vi "SCLN_Servers.vi"() -> (0 "Number of Servers":i32=1 min=1 max=7)   [LabVIEW 2015]
doc: "This VI activates as many servers as declared in the \ninitialization VI. A listener for each server is created\nand a server loop is entered to handle the client\nmessages."
uses:
  SCLN_RW_Select.ctl
  SCLN_INT32_Select.ctl
  SCLN_NOTIF_Select.ctl
panel:
  out "Port7":string
  out "Port6":string
  out "Port5":string
  out "Port4":string
  out "Port3":string
  out "Port2":string
  out "Port1":string
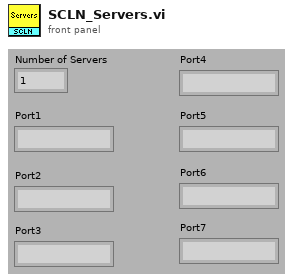
[diagram p1: front panel]
types:
  T1 = typedef "SCLN_INT32_Select.ctl" = enum16{"Max_Servers", "Max_Clients", "Total_Servers", "Total_Clients"}
  T2 = typedef "SCLN_RW_Select.ctl" = enum16{"Read", "Write"}
  T3 = typedef "SCLN_NOTIF_Select.ctl" = enum16{"Server1", "Server2", "Server3", "Server4", "Server5", "Server6", "Server7", "Client1", "Client2", "Client3", "Client4", "Client5", "Client6", "Client7", "Client8", "Client9", "Client10", "Shutdown", "Init_Ready"}
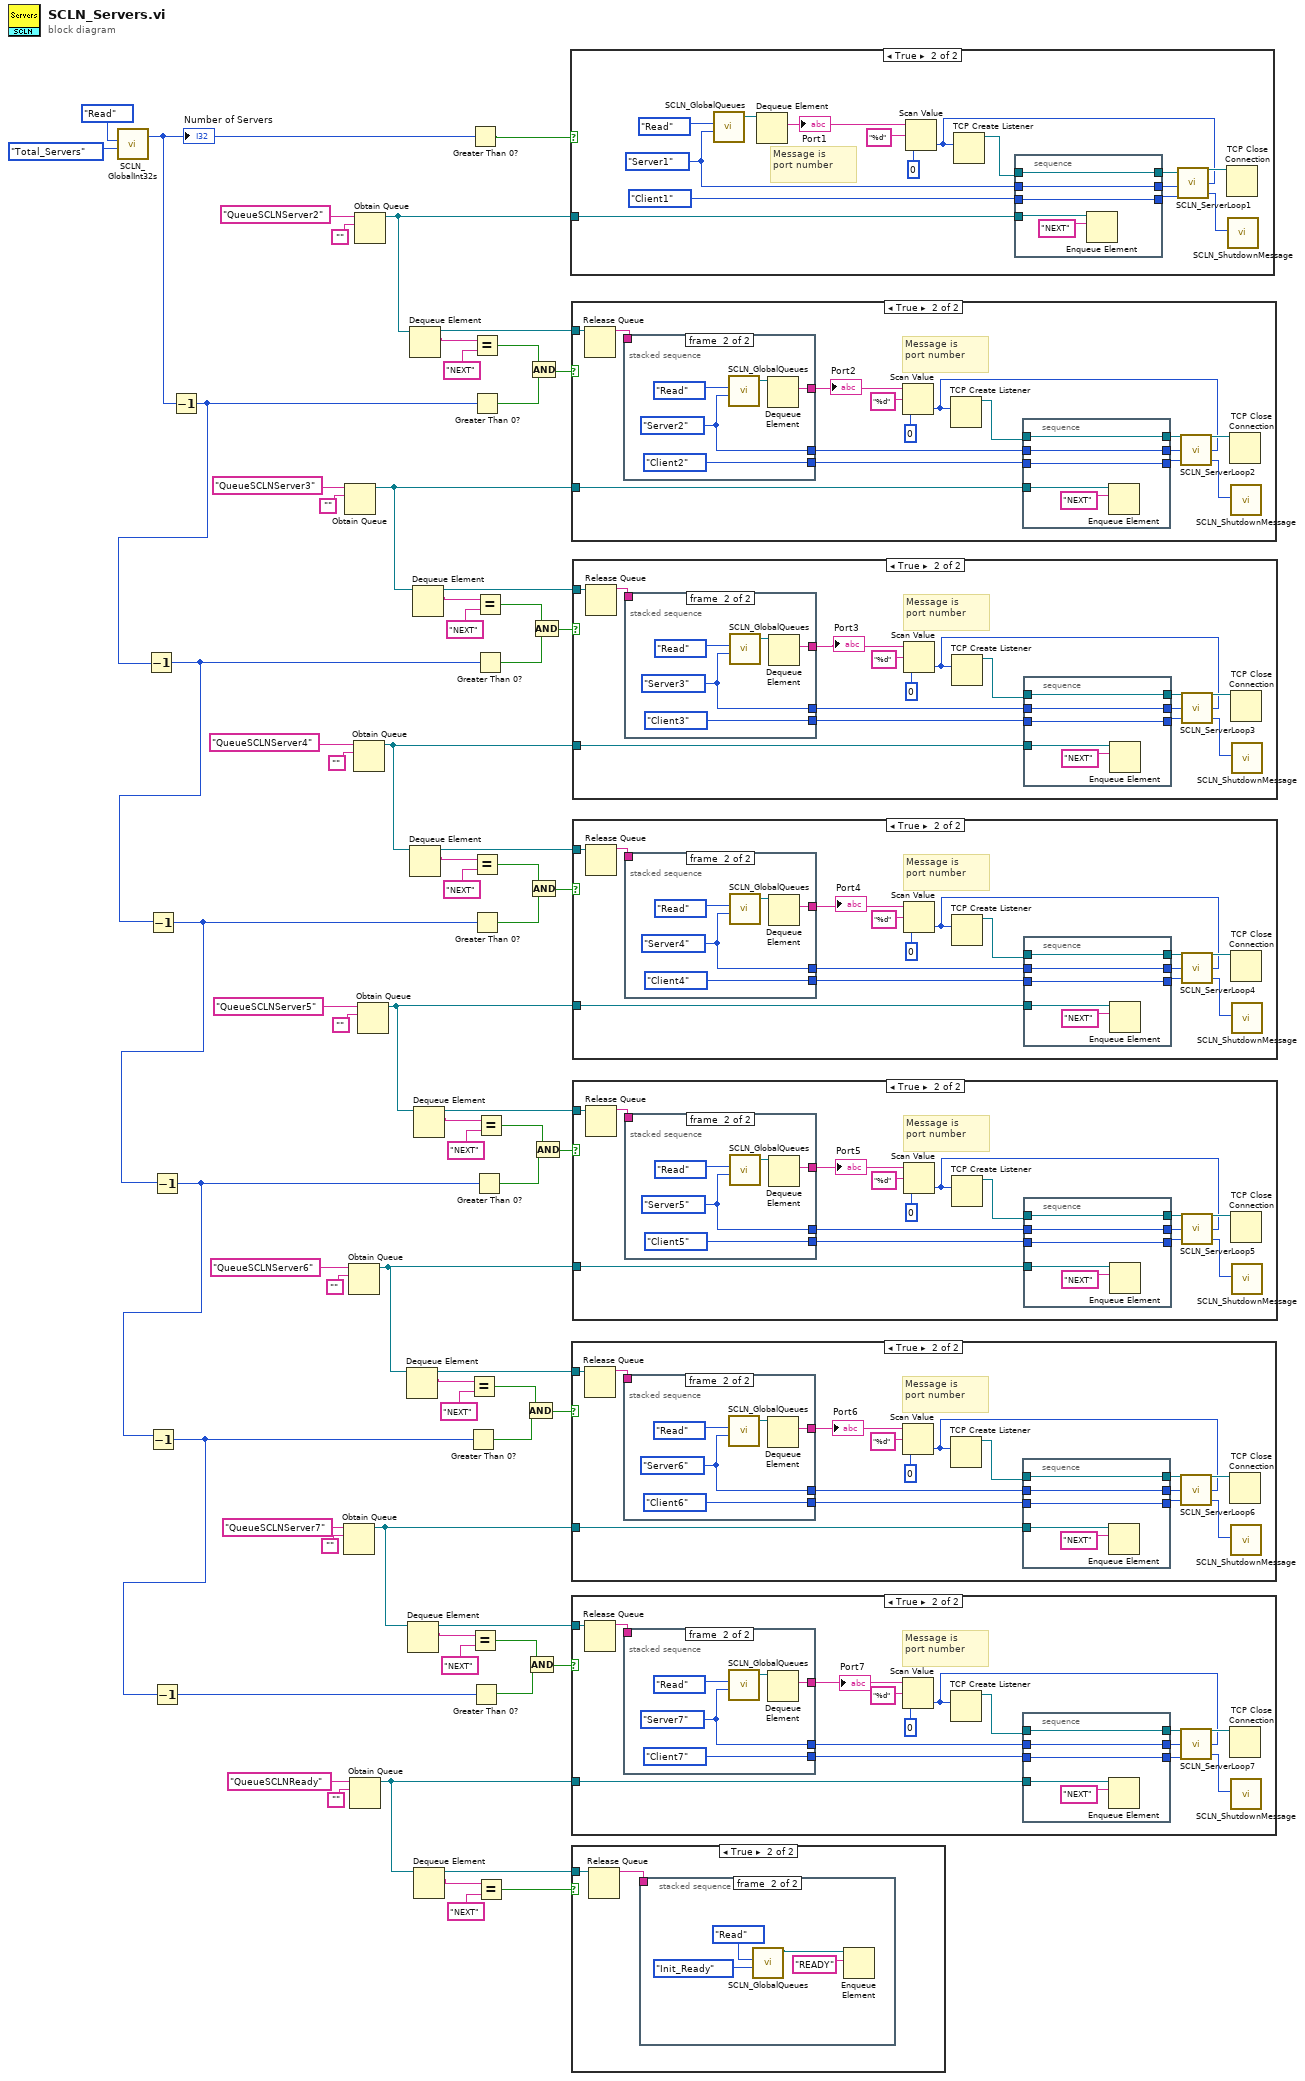
[diagram p0: block diagram]
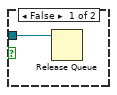
[diagram p2: hidden frame]
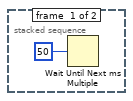
[diagram p3: hidden frame]
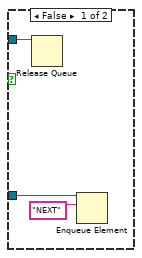
[diagram p4: hidden frame]
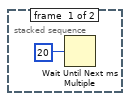
[diagram p5: hidden frame]
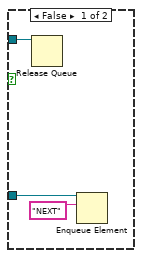
[diagram p6: hidden frame]
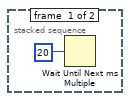
[diagram p7: hidden frame]
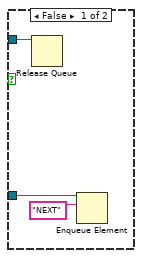
[diagram p8: hidden frame]
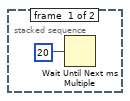
[diagram p9: hidden frame]
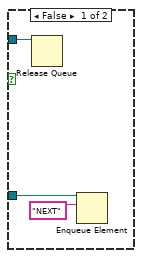
[diagram p10: hidden frame]
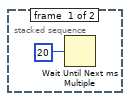
[diagram p11: hidden frame]
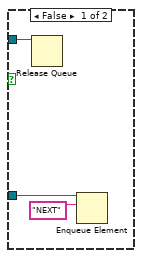
[diagram p12: hidden frame]
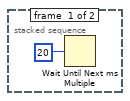
[diagram p13: hidden frame]
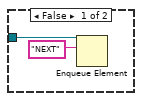
[diagram p14: hidden frame]
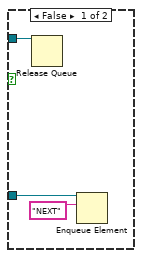
[diagram p15: hidden frame]
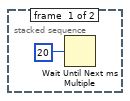
[diagram p16: hidden frame]
diagram:
  n1 = call "SCLN_GlobalInt32s.vi"("Element"=SCLN_INT32_Select."Total_Servers" ("GBL_INT32"), "Operation"=SCLN_RW_Select."Read" ("GBL_RW")) -> ("Read Value"=w70:i32)  [unwired: 2 in, 1 out]
  "Number of Servers" <- w70
  n2 = Decrement(x=w70) -> (x-1=w16:i32)
  n3 = Decrement(x=w16) -> (x-1=w15:i32)
  n4 = Decrement(x=w15) -> (x-1=w14:i32)
  n5 = Decrement(x=w14) -> (x-1=w13:i32)
  n6 = Decrement(x=w13) -> (x-1=w12:i32)
  n7 = Decrement(x=w12) -> (x-1=w69:i32)
  n8 = Obtain Queue(name (unnamed)="QueueSCLNServer7", element data type="") -> (queue out=w18:refnum<queue>)  [unwired: 3 in, 2 out]
  n9 = Obtain Queue(name (unnamed)="QueueSCLNServer3", element data type="") -> (queue out=w53:refnum<queue>)  [unwired: 3 in, 2 out]
  n10 = Obtain Queue(name (unnamed)="QueueSCLNServer6", element data type="") -> (queue out=w27:refnum<queue>)  [unwired: 3 in, 2 out]
  n11 = Obtain Queue(name (unnamed)="QueueSCLNReady", element data type="") -> (queue out=w5:refnum<queue>)  [unwired: 3 in, 2 out]
  n12 = Obtain Queue(name (unnamed)="QueueSCLNServer4", element data type="") -> (queue out=w44:refnum<queue>)  [unwired: 3 in, 2 out]
  n13 = Obtain Queue(name (unnamed)="QueueSCLNServer2", element data type="") -> (queue out=w64:refnum<queue>)  [unwired: 3 in, 2 out]
  n14 = Obtain Queue(name (unnamed)="QueueSCLNServer5", element data type="") -> (queue out=w35:refnum<queue>)  [unwired: 3 in, 2 out]
  n15 = Dequeue Element(queue=w27) -> (queue out=w25:refnum<queue>, element=w31:string)  [unwired: 2 in, 2 out]
  n16 = Dequeue Element(queue=w18) -> (queue out=w10:refnum<queue>, element=w21:string)  [unwired: 2 in, 2 out]
  n17 = Dequeue Element(queue=w64) -> (queue out=w60:refnum<queue>, element=w59:string)  [unwired: 2 in, 2 out]
  n18 = Dequeue Element(queue=w44) -> (queue out=w43:refnum<queue>, element=w47:string)  [unwired: 2 in, 2 out]
  n19 = Dequeue Element(queue=w53) -> (queue out=w51:refnum<queue>, element=w55:string)  [unwired: 2 in, 2 out]
  n20 = Dequeue Element(queue=w35) -> (queue out=w33:refnum<queue>, element=w40:string)  [unwired: 2 in, 2 out]
  n21 = Dequeue Element(queue=w5) -> (queue out=w3:refnum<queue>, element=w7:string)  [unwired: 2 in, 2 out]
  n22 = Greater Than 0?(x=w12) -> (x > 0?=w26:bool)
  n23 = Equal?(x=w31, y="NEXT") -> (x = y?=w29:bool)
  n24 = Greater Than 0?(x=w70) -> (x > 0?=w67:bool)
  n25 = Equal?(x=w21, y="NEXT") -> (x = y?=w19:bool)
  n26 = Greater Than 0?(x=w69) -> (x > 0?=w17:bool)
  n27 = Equal?(x=w59, y="NEXT") -> (x = y?=w2:bool)
  n28 = Greater Than 0?(x=w16) -> (x > 0?=w63:bool)
  n29 = Equal?(x=w47, y="NEXT") -> (x = y?=w48:bool)
  n30 = Greater Than 0?(x=w14) -> (x > 0?=w49:bool)
  n31 = Greater Than 0?(x=w13) -> (x > 0?=w37:bool)
  n32 = Equal?(x=w55, y="NEXT") -> (x = y?=w56:bool)
  n33 = Greater Than 0?(x=w15) -> (x > 0?=w57:bool)
  n34 = Equal?(x=w40, y="NEXT") -> (x = y?=w38:bool)
  n35 = Equal?(x=w7, y="NEXT") -> (x = y?=w4:bool)
  n36 = Compound Arithmetic op=AND(w29, w26) -> (w24:bool)
  n37 = Compound Arithmetic op=AND(w19, w17) -> (w11:bool)
  n38 = Compound Arithmetic op=AND(w2, w63) -> (w1:bool)
  n39 = Compound Arithmetic op=AND(w48, w49) -> (w42:bool)
  n40 = Compound Arithmetic op=AND(w56, w57) -> (w52:bool)
  n41 = Compound Arithmetic op=AND(w38, w37) -> (w36:bool)
  n42 = case shown="True" w67 {
    tunnel: w64 -> [w73 w74]
    frame False {
      n43 = Enqueue Element(queue=w73, element="NEXT") -> ()  [unwired: 2 in, 3 out]
    }
    frame True {
      w81 = SCLN_NOTIF_Select."Server1" ("Dome String Ctrl")
      # "Message is\nport number"
      n44 = call "SCLN_GlobalQueues.vi"("Element"=w81, "Operation"=SCLN_RW_Select."Read" ("GBL_RW")) -> ("Read QueueID"=w79:refnum<queue>)  [unwired: 6 in, 1 out]
      n45 = Dequeue Element(queue=w79) -> (element=w77:string)  [unwired: 2 in, 3 out]
      "Port1" <- w77
      n46 = Scan Value(string=w77, format string="%d", default (0 dbl)=0) -> (value=w76:i32)  [unwired: 1 out]
      n47 = TCP Create Listener(10:w76) -> (3:w82:refnum<k5>)  [unwired: 4 in, 2 out]
      n48 = stacked-sequence {
        tunnel: w82 -> [w93]
        tunnel: w81 -> [w92]
        tunnel: SCLN_NOTIF_Select."Client1" ("Dome String Ctrl") -> [w91]
        tunnel: [w93] -> w75
        tunnel: [w92] -> w78
        tunnel: [w91] -> w80
        tunnel: w74 -> [w90]
        frame #0 {
          n49 = Enqueue Element(queue=w90, element="NEXT") -> ()  [unwired: 2 in, 3 out]
        }
      }
      n50 = call "SCLN_ServerLoop1.vi"("Server Port"=w76, "Client Number"=w80, "Server Number"=w78, "TCP IN"=w75) -> ("Server Out"=w84:i32, "TCP OUT"=w85:refnum<k5>)
      n51 = TCP Close Connection(connection ID=w85) -> ()  [unwired: 2 in, 2 out]
      n52 = call "SCLN_ShutdownMessage.vi"("Server Number"=w84) -> ()
    }
  }
  n53 = case shown="True" w1 {
    tunnel: w53 -> [w95 w99]
    tunnel: w60 -> [w94 w100]
    frame False {
      n54 = Release Queue(queue=w94) -> ()  [unwired: 2 in, 3 out]
      n55 = Enqueue Element(queue=w95, element="NEXT") -> ()  [unwired: 2 in, 3 out]
    }
    frame True {
      # "Message is\nport number"
      n56 = Release Queue(queue=w100) -> (queue name=w97:string)  [unwired: 2 in, 2 out]
      n57 = stacked-sequence {
        tunnel: [_ SCLN_NOTIF_Select."Client2" ("Dome String Ctrl")] -> w107
        tunnel: [_ w115] -> w105
        tunnel: [_ w113] -> w98
        tunnel: w97 -> [_ _]
        frame #0 {
          n58 = Wait Until Next ms Multiple(millisecond multiple=20) -> ()  [unwired: 1 out]
        }
        frame #1 {
          w115 = SCLN_NOTIF_Select."Server2" ("Dome String Ctrl")
          n59 = call "SCLN_GlobalQueues.vi"("Element"=w115, "Operation"=SCLN_RW_Select."Read" ("GBL_RW")) -> ("Read QueueID"=w114:refnum<queue>)  [unwired: 6 in, 1 out]
          n60 = Dequeue Element(queue=w114) -> (element=w113:string)  [unwired: 2 in, 3 out]
        }
      }
      "Port2" <- w98
      n61 = Scan Value(string=w98, format string="%d", default (0 dbl)=0) -> (value=w102:i32)  [unwired: 1 out]
      n62 = TCP Create Listener(10:w102) -> (3:w106:refnum<k5>)  [unwired: 4 in, 2 out]
      n63 = stacked-sequence {
        tunnel: w106 -> [w122]
        tunnel: w105 -> [w121]
        tunnel: w107 -> [w120]
        tunnel: [w122] -> w101
        tunnel: [w121] -> w103
        tunnel: [w120] -> w104
        tunnel: w99 -> [w118]
        frame #0 {
          n64 = Enqueue Element(queue=w118, element="NEXT") -> ()  [unwired: 2 in, 3 out]
        }
      }
      n65 = call "SCLN_ServerLoop2.vi"("Server Port"=w102, "Client Number"=w104, "Server Number"=w103, "TCP IN"=w101) -> ("Server Out"=w108:i32, "TCP OUT"=w109:refnum<k5>)
      n66 = TCP Close Connection(connection ID=w109) -> ()  [unwired: 2 in, 2 out]
      n67 = call "SCLN_ShutdownMessage.vi"("Server Number"=w108) -> ()
    }
  }
  n68 = case shown="True" w24 {
    tunnel: w18 -> [w124 w129]
    tunnel: w25 -> [w123 w128]
    frame False {
      n69 = Release Queue(queue=w123) -> ()  [unwired: 2 in, 3 out]
      n70 = Enqueue Element(queue=w124, element="NEXT") -> ()  [unwired: 2 in, 3 out]
    }
    frame True {
      # "Message is\nport number"
      n71 = Release Queue(queue=w128) -> (queue name=w127:string)  [unwired: 2 in, 2 out]
      n72 = stacked-sequence {
        tunnel: [_ SCLN_NOTIF_Select."Client6" ("Dome String Ctrl")] -> w136
        tunnel: [_ w144] -> w134
        tunnel: [_ w142] -> w126
        tunnel: w127 -> [_ _]
        frame #0 {
          n73 = Wait Until Next ms Multiple(millisecond multiple=20) -> ()  [unwired: 1 out]
        }
        frame #1 {
          w144 = SCLN_NOTIF_Select."Server6" ("Dome String Ctrl")
          n74 = call "SCLN_GlobalQueues.vi"("Element"=w144, "Operation"=SCLN_RW_Select."Read" ("GBL_RW")) -> ("Read QueueID"=w143:refnum<queue>)  [unwired: 6 in, 1 out]
          n75 = Dequeue Element(queue=w143) -> (element=w142:string)  [unwired: 2 in, 3 out]
        }
      }
      "Port6" <- w126
      n76 = Scan Value(string=w126, format string="%d", default (0 dbl)=0) -> (value=w131:i32)  [unwired: 1 out]
      n77 = TCP Create Listener(10:w131) -> (3:w135:refnum<k5>)  [unwired: 4 in, 2 out]
      n78 = stacked-sequence {
        tunnel: w135 -> [w151]
        tunnel: w134 -> [w150]
        tunnel: w136 -> [w149]
        tunnel: [w151] -> w130
        tunnel: [w150] -> w132
        tunnel: [w149] -> w133
        tunnel: w129 -> [w147]
        frame #0 {
          n79 = Enqueue Element(queue=w147, element="NEXT") -> ()  [unwired: 2 in, 3 out]
        }
      }
      n80 = call "SCLN_ServerLoop6.vi"("Server Port"=w131, "Client Number"=w133, "Server Number"=w132, "TCP IN"=w130) -> ("Server Out"=w137:i32, "TCP OUT"=w138:refnum<k5>)
      n81 = TCP Close Connection(connection ID=w138) -> ()  [unwired: 2 in, 2 out]
      n82 = call "SCLN_ShutdownMessage.vi"("Server Number"=w137) -> ()
    }
  }
  n83 = case shown="True" w11 {
    tunnel: w5 -> [w153 w160]
    tunnel: w10 -> [w152 w159]
    frame False {
      n84 = Release Queue(queue=w152) -> ()  [unwired: 2 in, 3 out]
      n85 = Enqueue Element(queue=w153, element="NEXT") -> ()  [unwired: 2 in, 3 out]
    }
    frame True {
      # "Message is\nport number"
      n86 = Release Queue(queue=w159) -> (queue name=w158:string)  [unwired: 2 in, 2 out]
      n87 = stacked-sequence {
        tunnel: [_ SCLN_NOTIF_Select."Client7" ("Dome String Ctrl")] -> w165
        tunnel: [_ w173] -> w163
        tunnel: [_ w171] -> w155
        tunnel: w158 -> [_ _]
        frame #0 {
          n88 = Wait Until Next ms Multiple(millisecond multiple=20) -> ()  [unwired: 1 out]
        }
        frame #1 {
          w173 = SCLN_NOTIF_Select."Server7" ("Dome String Ctrl")
          n89 = call "SCLN_GlobalQueues.vi"("Element"=w173, "Operation"=SCLN_RW_Select."Read" ("GBL_RW")) -> ("Read QueueID"=w172:refnum<queue>)  [unwired: 6 in, 1 out]
          n90 = Dequeue Element(queue=w172) -> (element=w171:string)  [unwired: 2 in, 3 out]
        }
      }
      "Port7" <- w155
      n91 = Scan Value(string=w155, format string="%d", default (0 dbl)=0) -> (value=w157:i32)  [unwired: 1 out]
      n92 = TCP Create Listener(10:w157) -> (3:w164:refnum<k5>)  [unwired: 4 in, 2 out]
      n93 = stacked-sequence {
        tunnel: w164 -> [w180]
        tunnel: w163 -> [w179]
        tunnel: w165 -> [w178]
        tunnel: [w180] -> w161
        tunnel: [w179] -> w162
        tunnel: [w178] -> w156
        tunnel: w160 -> [w176]
        frame #0 {
          n94 = Enqueue Element(queue=w176, element="NEXT") -> ()  [unwired: 2 in, 3 out]
        }
      }
      n95 = call "SCLN_ServerLoop7.vi"("Server Port"=w157, "Client Number"=w156, "Server Number"=w162, "TCP IN"=w161) -> ("Server Out"=w166:i32, "TCP OUT"=w167:refnum<k5>)
      n96 = TCP Close Connection(connection ID=w167) -> ()  [unwired: 2 in, 2 out]
      n97 = call "SCLN_ShutdownMessage.vi"("Server Number"=w166) -> ()
    }
  }
  n98 = case shown="True" w4 {
    tunnel: w3 -> [w181 w183]
    frame False {
      n99 = Release Queue(queue=w181) -> ()  [unwired: 2 in, 3 out]
    }
    frame True {
      n100 = Release Queue(queue=w183) -> (queue name=w182:string)  [unwired: 2 in, 2 out]
      n101 = stacked-sequence {
        tunnel: w182 -> [_ _]
        frame #0 {
          n102 = Wait Until Next ms Multiple(millisecond multiple=50) -> ()  [unwired: 1 out]
        }
        frame #1 {
          n103 = call "SCLN_GlobalQueues.vi"("Element"=SCLN_NOTIF_Select."Init_Ready" ("Dome String Ctrl"), "Operation"=SCLN_RW_Select."Read" ("GBL_RW")) -> ("Read QueueID"=w187:refnum<queue>)  [unwired: 6 in, 1 out]
          n104 = Enqueue Element(queue=w187, element="READY") -> ()  [unwired: 2 in, 3 out]
        }
      }
    }
  }
  n105 = case shown="True" w52 {
    tunnel: w44 -> [w190 w195]
    tunnel: w51 -> [w189 w194]
    frame False {
      n106 = Release Queue(queue=w189) -> ()  [unwired: 2 in, 3 out]
      n107 = Enqueue Element(queue=w190, element="NEXT") -> ()  [unwired: 2 in, 3 out]
    }
    frame True {
      # "Message is\nport number"
      n108 = Release Queue(queue=w194) -> (queue name=w192:string)  [unwired: 2 in, 2 out]
      n109 = stacked-sequence {
        tunnel: [_ SCLN_NOTIF_Select."Client3" ("Dome String Ctrl")] -> w202
        tunnel: [_ w210] -> w200
        tunnel: [_ w208] -> w193
        tunnel: w192 -> [_ _]
        frame #0 {
          n110 = Wait Until Next ms Multiple(millisecond multiple=20) -> ()  [unwired: 1 out]
        }
        frame #1 {
          w210 = SCLN_NOTIF_Select."Server3" ("Dome String Ctrl")
          n111 = call "SCLN_GlobalQueues.vi"("Element"=w210, "Operation"=SCLN_RW_Select."Read" ("GBL_RW")) -> ("Read QueueID"=w209:refnum<queue>)  [unwired: 6 in, 1 out]
          n112 = Dequeue Element(queue=w209) -> (element=w208:string)  [unwired: 2 in, 3 out]
        }
      }
      "Port3" <- w193
      n113 = Scan Value(string=w193, format string="%d", default (0 dbl)=0) -> (value=w197:i32)  [unwired: 1 out]
      n114 = TCP Create Listener(10:w197) -> (3:w201:refnum<k5>)  [unwired: 4 in, 2 out]
      n115 = stacked-sequence {
        tunnel: w201 -> [w217]
        tunnel: w200 -> [w216]
        tunnel: w202 -> [w215]
        tunnel: [w217] -> w196
        tunnel: [w216] -> w198
        tunnel: [w215] -> w199
        tunnel: w195 -> [w213]
        frame #0 {
          n116 = Enqueue Element(queue=w213, element="NEXT") -> ()  [unwired: 2 in, 3 out]
        }
      }
      n117 = call "SCLN_ServerLoop3.vi"("Server Port"=w197, "Client Number"=w199, "Server Number"=w198, "TCP IN"=w196) -> ("Server Out"=w203:i32, "TCP OUT"=w204:refnum<k5>)
      n118 = TCP Close Connection(connection ID=w204) -> ()  [unwired: 2 in, 2 out]
      n119 = call "SCLN_ShutdownMessage.vi"("Server Number"=w203) -> ()
    }
  }
  n120 = case shown="True" w42 {
    tunnel: w35 -> [w219 w224]
    tunnel: w43 -> [w218 w223]
    frame False {
      n121 = Release Queue(queue=w218) -> ()  [unwired: 2 in, 3 out]
      n122 = Enqueue Element(queue=w219, element="NEXT") -> ()  [unwired: 2 in, 3 out]
    }
    frame True {
      # "Message is\nport number"
      n123 = Release Queue(queue=w223) -> (queue name=w221:string)  [unwired: 2 in, 2 out]
      n124 = stacked-sequence {
        tunnel: [_ SCLN_NOTIF_Select."Client4" ("Dome String Ctrl")] -> w231
        tunnel: [_ w239] -> w229
        tunnel: [_ w237] -> w222
        tunnel: w221 -> [_ _]
        frame #0 {
          n125 = Wait Until Next ms Multiple(millisecond multiple=20) -> ()  [unwired: 1 out]
        }
        frame #1 {
          w239 = SCLN_NOTIF_Select."Server4" ("Dome String Ctrl")
          n126 = call "SCLN_GlobalQueues.vi"("Element"=w239, "Operation"=SCLN_RW_Select."Read" ("GBL_RW")) -> ("Read QueueID"=w238:refnum<queue>)  [unwired: 6 in, 1 out]
          n127 = Dequeue Element(queue=w238) -> (element=w237:string)  [unwired: 2 in, 3 out]
        }
      }
      "Port4" <- w222
      n128 = Scan Value(string=w222, format string="%d", default (0 dbl)=0) -> (value=w226:i32)  [unwired: 1 out]
      n129 = TCP Create Listener(10:w226) -> (3:w230:refnum<k5>)  [unwired: 4 in, 2 out]
      n130 = stacked-sequence {
        tunnel: w230 -> [w246]
        tunnel: w229 -> [w245]
        tunnel: w231 -> [w244]
        tunnel: [w246] -> w225
        tunnel: [w245] -> w227
        tunnel: [w244] -> w228
        tunnel: w224 -> [w242]
        frame #0 {
          n131 = Enqueue Element(queue=w242, element="NEXT") -> ()  [unwired: 2 in, 3 out]
        }
      }
      n132 = call "SCLN_ServerLoop4.vi"("Server Port"=w226, "Client Number"=w228, "Server Number"=w227, "TCP IN"=w225) -> ("Server Out"=w232:i32, "TCP OUT"=w233:refnum<k5>)
      n133 = TCP Close Connection(connection ID=w233) -> ()  [unwired: 2 in, 2 out]
      n134 = call "SCLN_ShutdownMessage.vi"("Server Number"=w232) -> ()
    }
  }
  n135 = case shown="True" w36 {
    tunnel: w27 -> [w248 w253]
    tunnel: w33 -> [w247 w252]
    frame False {
      n136 = Release Queue(queue=w247) -> ()  [unwired: 2 in, 3 out]
      n137 = Enqueue Element(queue=w248, element="NEXT") -> ()  [unwired: 2 in, 3 out]
    }
    frame True {
      # "Message is\nport number"
      n138 = Release Queue(queue=w252) -> (queue name=w250:string)  [unwired: 2 in, 2 out]
      n139 = stacked-sequence {
        tunnel: [_ SCLN_NOTIF_Select."Client5" ("Dome String Ctrl")] -> w260
        tunnel: [_ w268] -> w258
        tunnel: [_ w266] -> w251
        tunnel: w250 -> [_ _]
        frame #0 {
          n140 = Wait Until Next ms Multiple(millisecond multiple=20) -> ()  [unwired: 1 out]
        }
        frame #1 {
          w268 = SCLN_NOTIF_Select."Server5" ("Dome String Ctrl")
          n141 = call "SCLN_GlobalQueues.vi"("Element"=w268, "Operation"=SCLN_RW_Select."Read" ("GBL_RW")) -> ("Read QueueID"=w267:refnum<queue>)  [unwired: 6 in, 1 out]
          n142 = Dequeue Element(queue=w267) -> (element=w266:string)  [unwired: 2 in, 3 out]
        }
      }
      "Port5" <- w251
      n143 = Scan Value(string=w251, format string="%d", default (0 dbl)=0) -> (value=w255:i32)  [unwired: 1 out]
      n144 = TCP Create Listener(10:w255) -> (3:w259:refnum<k5>)  [unwired: 4 in, 2 out]
      n145 = stacked-sequence {
        tunnel: w259 -> [w275]
        tunnel: w258 -> [w274]
        tunnel: w260 -> [w273]
        tunnel: [w275] -> w254
        tunnel: [w274] -> w256
        tunnel: [w273] -> w257
        tunnel: w253 -> [w271]
        frame #0 {
          n146 = Enqueue Element(queue=w271, element="NEXT") -> ()  [unwired: 2 in, 3 out]
        }
      }
      n147 = call "SCLN_ServerLoop5.vi"("Server Port"=w255, "Client Number"=w257, "Server Number"=w256, "TCP IN"=w254) -> ("Server Out"=w261:i32, "TCP OUT"=w262:refnum<k5>)
      n148 = TCP Close Connection(connection ID=w262) -> ()  [unwired: 2 in, 2 out]
      n149 = call "SCLN_ShutdownMessage.vi"("Server Number"=w261) -> ()
    }
  }
